vi "runscenario calculate relative timestamps.vi"(1 "Time Stamp (now)":timestamp) -> (0 "UTC Relative Timestamps":T1)   [LabVIEW 2011]
panel:
  out "Year Begin":timestamp
  out "Year Prior Begin":timestamp
  out "Month Begin":timestamp
  out "Month Prior Begin":timestamp
  out "Week Prior Begin":timestamp
  out "Week Begin":timestamp
  out "Day Prior Begin":timestamp
  out "Day End":timestamp
  out "Day Begin":timestamp
  # "Use below for debugging...\n  Note all times are STANDARD (so DST = 0) and this display\n  will depend on your PC's current local time zone."
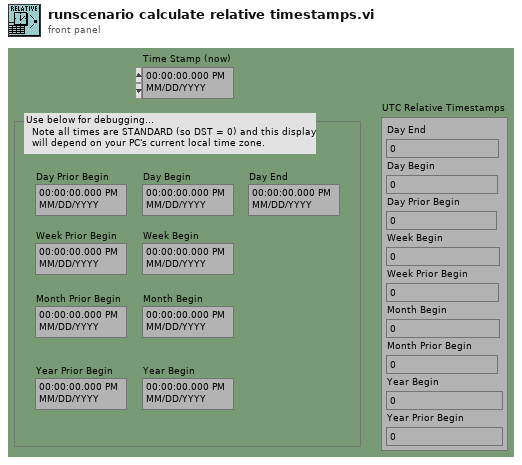
[diagram p1: front panel]
types:
  T1 = cluster{"Day End":dbl, "Day Begin":dbl, "Day Prior Begin":dbl, "Week Begin":dbl, "Week Prior Begin":dbl, "Month Begin":dbl, "Month Prior Begin":dbl, "Year Begin":dbl, "Year Prior Begin":dbl}
  T2 = cluster{"Today End":dbl, "Today Begin":dbl, "Yesterday Begin":dbl, "Week Begin":dbl, "Week Prior Begin":dbl, "Month Begin":dbl, "Month Prior Begin":dbl, "Year Begin":dbl, "Year Prior Begin":dbl}
  T3 = typedef "LVDateTimeRec.ctl" = cluster{"fractional second":dbl, "second":i32, "minute":i32, "hour":i32, "day of month":i32, "month":i32, "year":i32, "day of week":i32, "day of year":i32, "DST":i32}
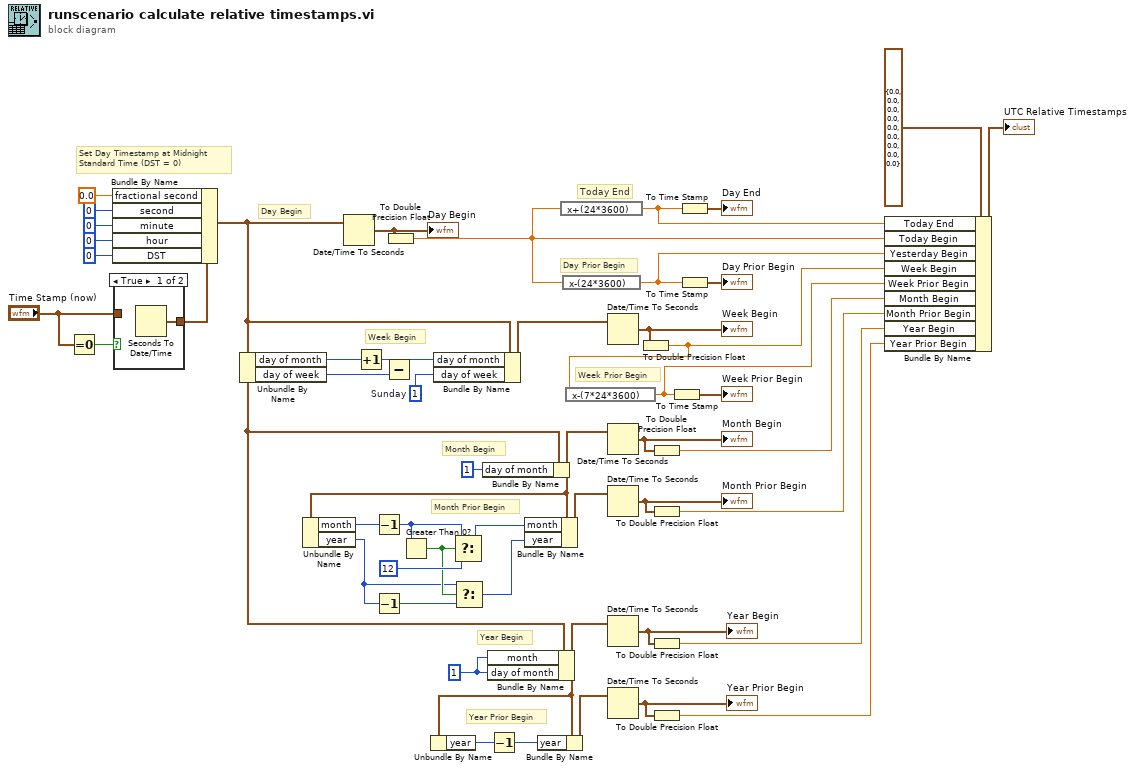
[diagram p0: block diagram]
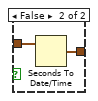
[diagram p2: hidden frame]
diagram:
  w2 = 1 ("day of month")
  w41 = 1  # Sunday
  # "Year Prior Begin"
  # "Year Begin"
  # "Month Prior Begin"
  # "Month Begin"
  # "Week Prior Begin"
  # "Week Begin"
  # "Day Prior Begin"
  # "Today End"
  # "Day Begin"
  # "Set Day Timestamp at Midnight \nStandard Time (DST = 0)"
  n1 = Equal To 0?(x="Time Stamp (now)") -> (x = 0?=w6:bool)
  n2 = case shown="True" w6 {
    tunnel: [w52 w54] -> w51
    tunnel: "Time Stamp (now)" -> [_ w53]
    frame True {
      n3 = Seconds To Date/Time() -> (date time rec=w52:T3)  [unwired: 2 out]
    }
    frame False {
      n4 = Seconds To Date/Time(time stamp (now)=w53) -> (date time rec=w54:T3)  [unwired: 1 out]
    }
  }
  n5 = Bundle By Name(cluster=w51, "fractional second"=0.0, "second"=0, "minute"=0, "hour"=0, "DST"=0) -> (w4:T3)
  n6 = Unbundle By Name(w4) -> ("day of month"=w40:i32, "day of week"=w38:i32)
  n7 = Date/Time To Seconds(2:w4) -> (0:w9:timestamp)  [unwired: 1 out]
  "Day Begin" <- w9
  n8 = Increment(x=w40) -> (x+1=w39:i32)
  n9 = Subtract(x=w39, y=w38) -> (x-y=w37:i32)
  n10 = To Double Precision Float(number=w9) -> (double precision float=w8:dbl)
  n11 = Bundle By Name(cluster=w4, "day of month"=w37, "day of week"=w41) -> (w42:T3)
  n12 = Bundle By Name(cluster=w4, "day of month"=1) -> (w29:T3)
  n13 = Unbundle By Name(w29) -> ("month"=w30:i32, "year"=w24:i32)
  n14 = Decrement(x=w30) -> (x-1=w28:i32)
  n15 = Decrement(x=w24) -> (x-1=w23:i32)
  n16 = Greater Than 0?(x=w28) -> (x > 0?=w25:bool)
  n17 = Select(t=w28, s=w25, f=12) -> (s? t:f=w27:i32)
  n18 = Select(t=w24, s=w25, f=w23) -> (s? t:f=w22:i32)
  n19 = Bundle By Name(cluster=w4, "month"=w2, "day of month"=w2) -> (w3:T3)
  n20 = Unbundle By Name(w3) -> ("year"=w21:i32)
  n21 = Decrement(x=w21) -> (x-1=w7:i32)
  n22 = Bundle By Name(cluster=w29, "month"=w27, "year"=w22) -> (w31:T3)
  n23 = Bundle By Name(cluster=w3, "year"=w7) -> (w20:T3)
  n24 = expression code="x+(24*3600)"(w8) -> (w33:dbl)
  n25 = expression code="x-(24*3600)"(w8) -> (w46:dbl)
  n26 = Date/Time To Seconds(2:w42) -> (0:w18:timestamp)  [unwired: 1 out]
  "Week Begin" <- w18
  n27 = Date/Time To Seconds(2:w29) -> (0:w17:timestamp)  [unwired: 1 out]
  "Month Begin" <- w17
  n28 = Date/Time To Seconds(2:w31) -> (0:w15:timestamp)  [unwired: 1 out]
  "Month Prior Begin" <- w15
  n29 = Date/Time To Seconds(2:w3) -> (0:w13:timestamp)  [unwired: 1 out]
  "Year Begin" <- w13
  n30 = Date/Time To Seconds(2:w20) -> (0:w11:timestamp)  [unwired: 1 out]
  "Year Prior Begin" <- w11
  n31 = To Double Precision Float(number=w18) -> (double precision float=w19:dbl)
  n32 = expression code="x-(7*24*3600)"(w19) -> (w35:dbl)
  n33 = To Double Precision Float(number=w17) -> (double precision float=w16:dbl)
  n34 = To Double Precision Float(number=w15) -> (double precision float=w14:dbl)
  n35 = To Double Precision Float(number=w13) -> (double precision float=w12:dbl)
  n36 = To Double Precision Float(number=w11) -> (double precision float=w10:dbl)
  n37 = To Time Stamp(1:w35) -> (0:→"Week Prior Begin":timestamp)
  n38 = To Time Stamp(1:w33) -> (0:→"Day End":timestamp)
  n39 = To Time Stamp(1:w46) -> (0:→"Day Prior Begin":timestamp)
  n40 = Bundle By Name(cluster=T2 {"Today End"=0.0, "Today Begin"=0.0, "Yesterday Begin"=0.0, "Week Begin"=0.0, "Week Prior Begin"=0.0, "Month Begin"=0.0, "Month Prior Begin"=0.0, "Year Begin"=0.0, "Year Prior Begin"=0.0} ("Relative Timestamps"), "Today End"=w33, "Today Begin"=w8, "Yesterday Begin"=w46, "Week Begin"=w19, "Week Prior Begin"=w35, "Month Begin"=w16, "Month Prior Begin"=w14, "Year Begin"=w12, "Year Prior Begin"=w10) -> (→"UTC Relative Timestamps":T2)
